vi "axis to position value.vi"(6 "Init Y":dbl=100.0, 9 "Init Z":dbl, 10 "axis info":T1, 11 "Init X":dbl) -> (1 "Y":dbl, 2 "OUT xyz":cluster{"X":i16, "Y":i16, "Z":i16}, 3 "X":dbl, 4 "Z":dbl)   [LabVIEW 2015]
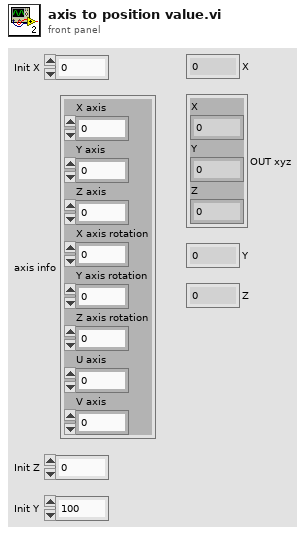
[diagram p1: front panel]
types:
  T1 = cluster{"X axis":i32, "Y axis":i32, "Z axis":i32, "X axis rotation":i32, "Y axis rotation":i32, "Z axis rotation":i32, "U axis":i32, "V axis":i32}
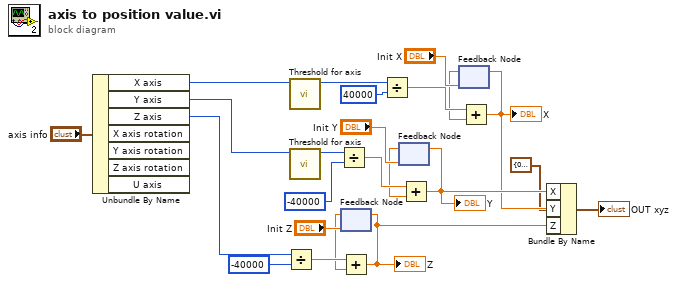
[diagram p0: block diagram]
diagram:
  n1 = Unbundle By Name("axis info") -> ("X axis"=w15:i32, "Y axis"=w17:i32, "Z axis"=w5:i32)  [unwired: 4 out]
  n2 = Divide(x=w5, y=-40000) -> (x/y=w11:dbl)
  n3 = call "Threshold for axis.vi"("X axis"=w15) -> ("Numeric"=w16:i32)  [unwired: 10 in]
  n4 = call "Threshold for axis.vi"("X axis"=w17) -> ("Numeric"=w18:i32)  [unwired: 10 in]
  n5 = Divide(x=w18, y=-40000) -> (x/y=w10:dbl)
  n6 = feedback #1("Init Z") -> (w8:dbl)
  n7 = Add(x=w11, y=w8) -> (x+y=w20:dbl)
  "Z" <- w20
  n8 = feedback-in #1(w20) -> ()
  n9 = Divide(x=w16, y=40000) -> (x/y=w9:dbl)
  n10 = feedback #2("Init Y") -> (w7:dbl)
  n11 = Add(x=w10, y=w7) -> (x+y=w22:dbl)
  "Y" <- w22
  n12 = feedback-in #2(w22) -> ()
  n13 = feedback #3("Init X") -> (w6:dbl)
  n14 = Add(x=w9, y=w6) -> (x+y=w21:dbl)
  "X" <- w21
  n15 = feedback-in #3(w21) -> ()
  n16 = Bundle By Name(cluster=cluster{"X":i16, "Y":i16, "Z":i16} {"X"=0, "Y"=0, "Z"=0} ("input cluster"), "X"=w22, "Y"=w21, "Z"=w20) -> (→"OUT xyz":cluster{"X":i16, "Y":i16, "Z":i16})
